vi "Catalytic Methanation #1.vi"() -> ()   [LabVIEW 2017]
uses:
  Halt S&THx.vi
  <vilib>/addons/control/pid/pid.llb/PID Advanced (DBL).vi
  <vilib>/addons/control/pid/NI_PID_pid.lvlib
panel:
  out "Heater Power Confirmed":bool
  in  "Td (Pressure)":dbl
  in  "Ti (Pressure)":dbl=0.01
  in  "Kc (Pressure)":dbl=-5.0
  in  "Td (Heater)":dbl caption="(min)"
  in  "Ti (Heater)":dbl=5.0 caption="(min)"
  in  "Kc (Heater)":dbl=1.0
  in  "GC Sample Path":enum32{"Reactor Feed", "Reactor Exhaust"}(radio)=enum."Reactor Exhaust"
  out "He Flowrate (SCCM)":dbl format="%.1f"
  out "H2 Flowrate (SCCM)":dbl format="%.2f"
  out "CO2 Flowrate (SCCM)":dbl format="%.2f"
  in  "He Setpoint (SCCM)":dbl min=0.0 max=200.0 format="%.1f"
  in  "H2 Setpoint (SCCM)":dbl min=0.0 max=50.0 format="%.2f"
  in  "Heater Switch":bool
  in  "CO2 Setpoint (SCCM)":dbl min=0.0 max=10.0 format="%.2f"
  in  "Temperature Setpoint (C)":dbl=20.0 min=0.0 max=325.0 format="%.1f"
  out "Reator Temperature (C)":dbl format="%.2f"
  out "Heater Output (%)":dbl(slide) scale=0.0..100.0
  in  "Manual Control Override (Temperature)":bool=TRUE
  in  "Set Manual Valve Heater Output (Temperature)":dbl(slide) scale=0.0..100.0
  in  "Reactor Pressure  Setpoint (psia)":dbl=18.4 min=0.0 max=30.0 format="%.1f"
  out "Reactor Pressure (psia)":dbl format="%.1f"
  out "Pressure Control Valve (%)":dbl(slide) scale=0.0..100.0
  in  "Manual Control Override (Pressure)":bool=TRUE
  in  "Set Manual Valve Position (Pressure)":dbl(slide)=50.0 scale=0.0..100.0
  in  "stop":bool
  out "Data Point Count":i32
  in  "Specify Time between Data Points (sec)":dbl=1.0
  in  "Cancel Data Collection":bool
  in  "Specify number of data points":i16=1
  in  "Enable 4":bool
  out "Saving Data 4":bool
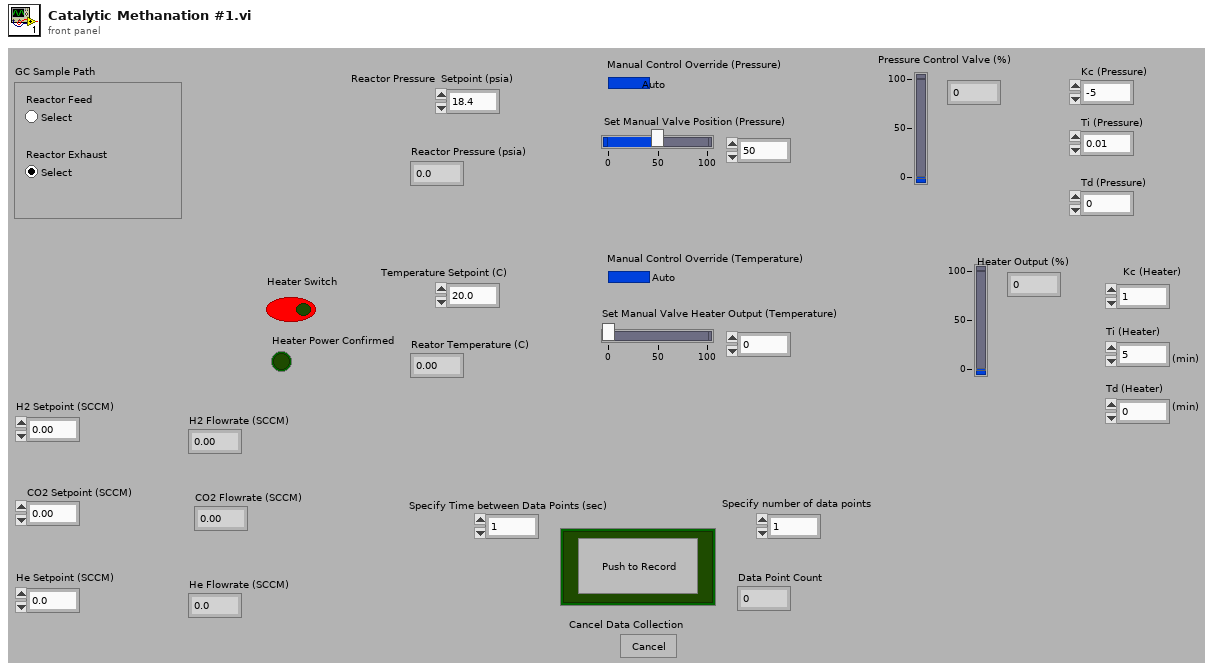
[diagram p1: front panel]
types:
  T1 = cluster{"Kc (Heater)":dbl, "Ti (Heater)":dbl, "Td (Heater)":dbl}
  T2 = cluster{"Kc (Pressure)":dbl, "Ti (Pressure)":dbl, "Td (Pressure)":dbl}
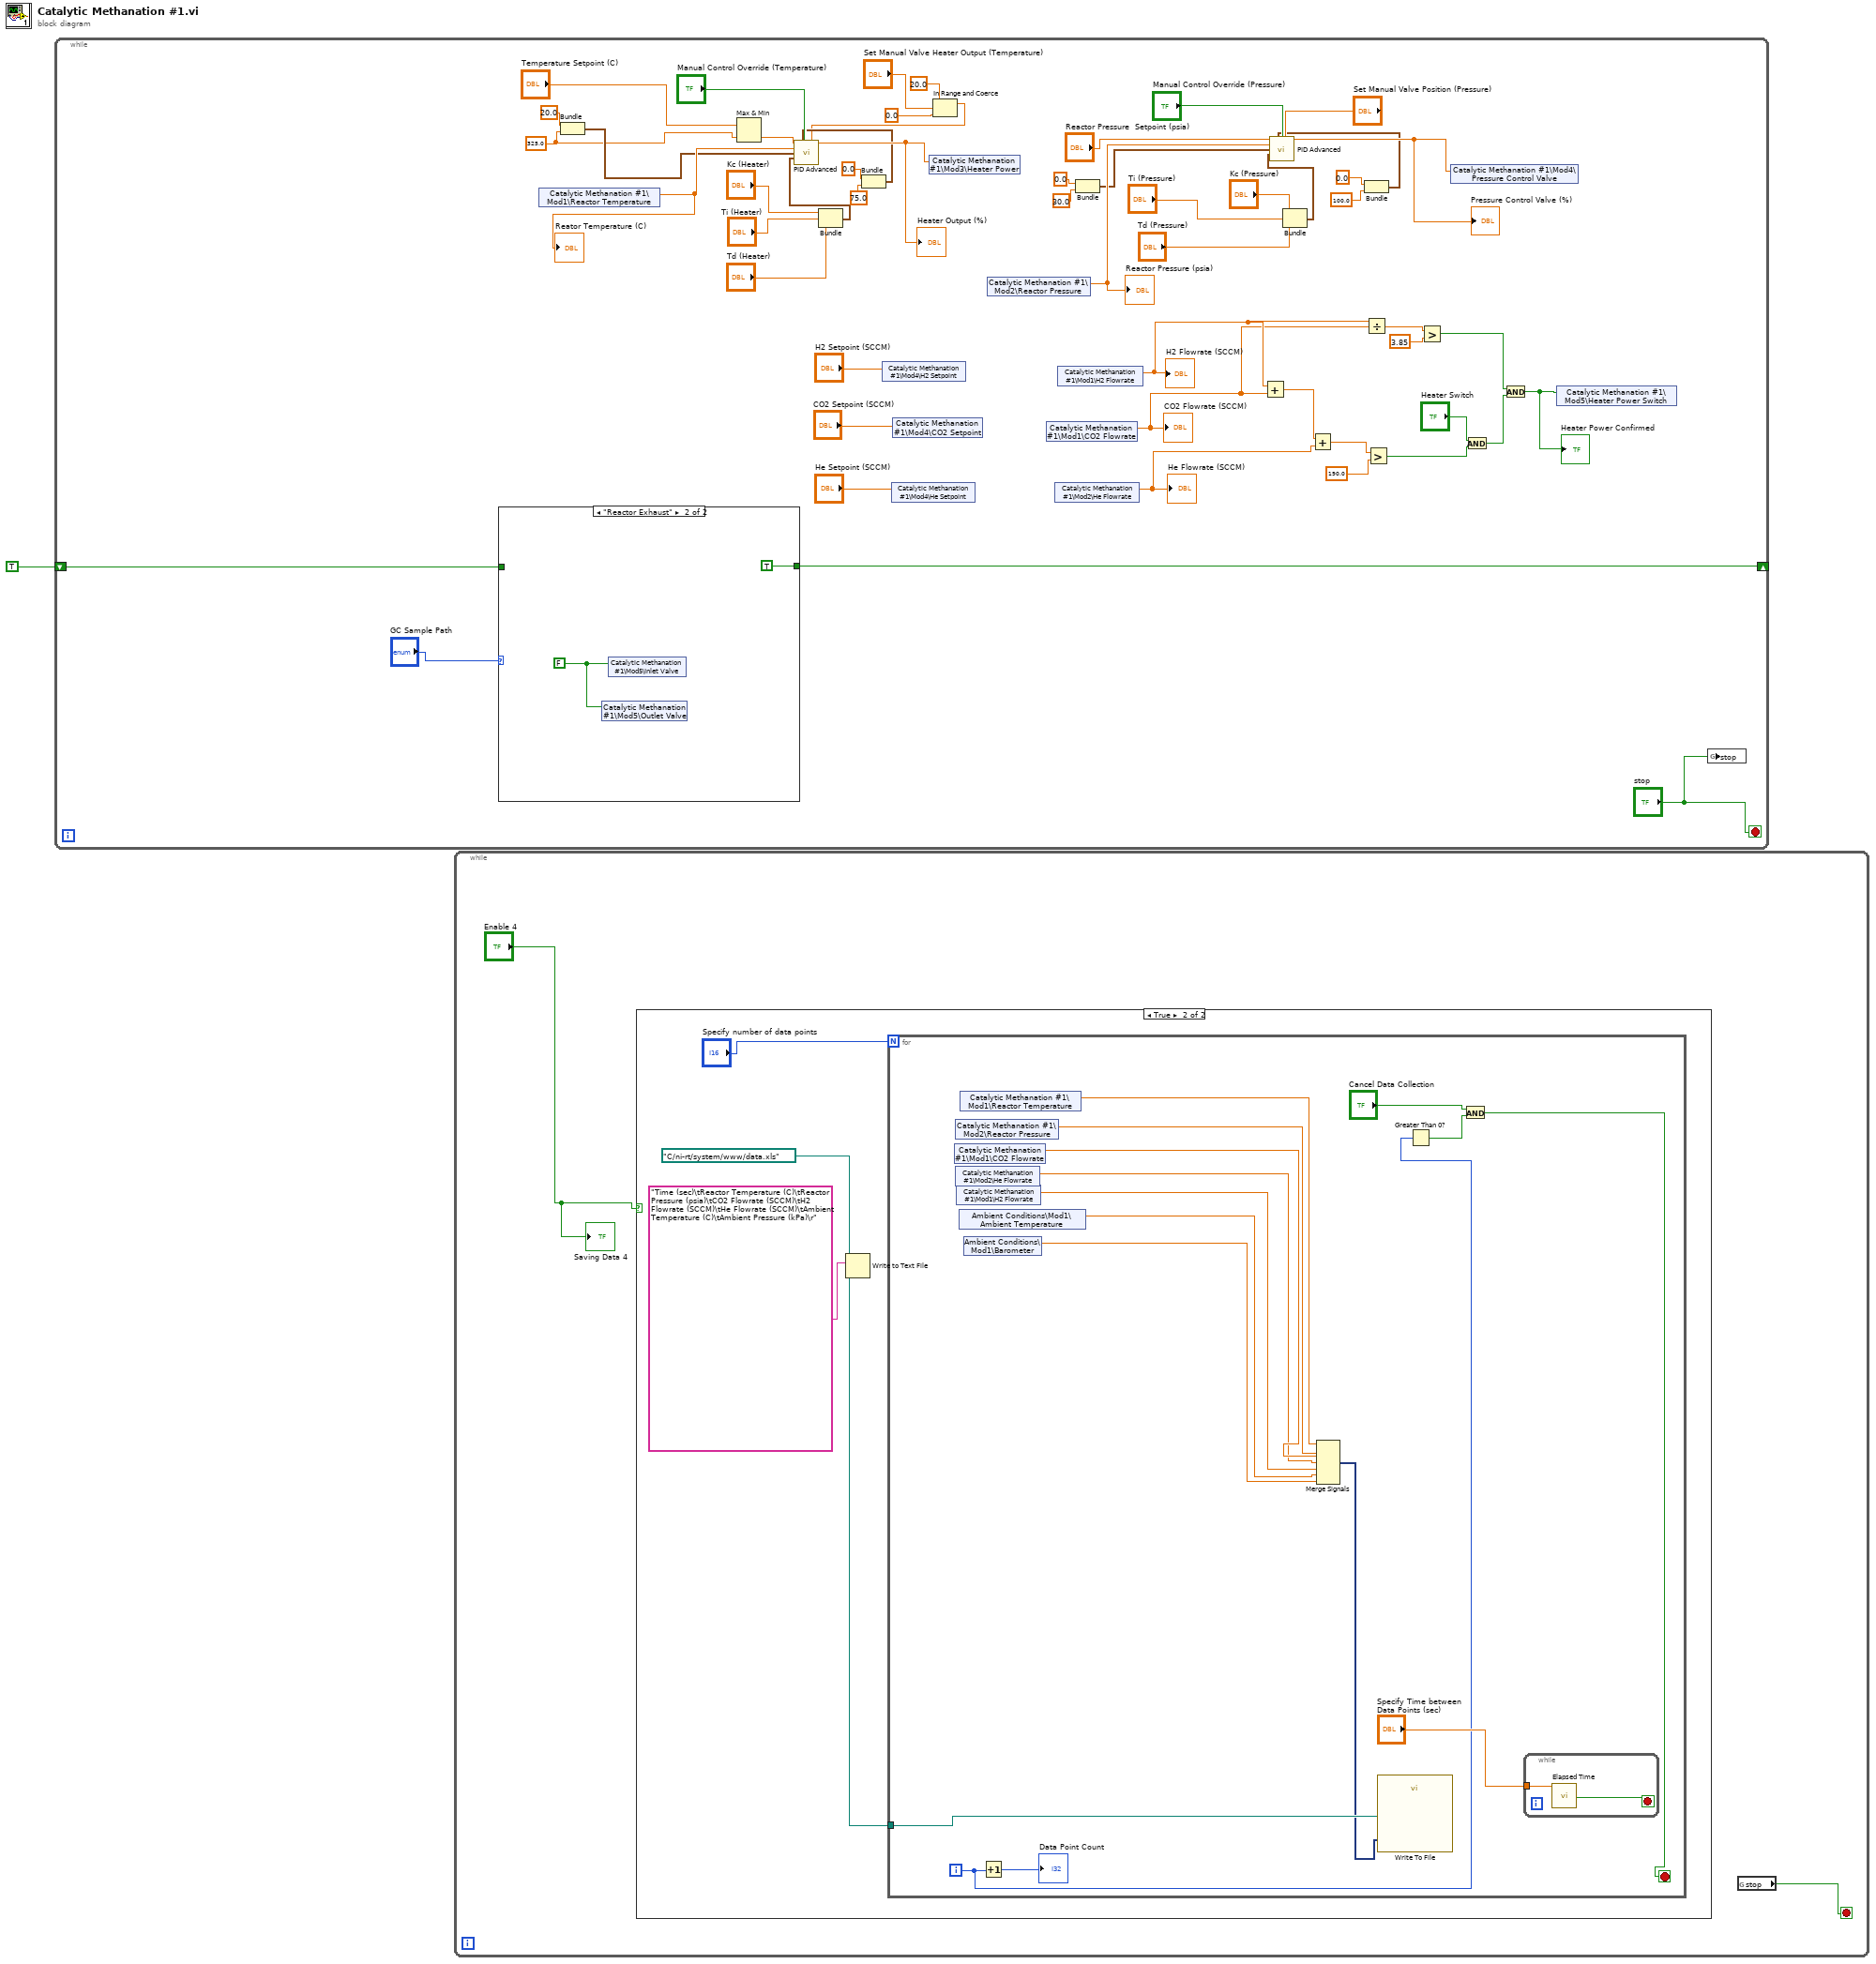
[diagram p0: block diagram]
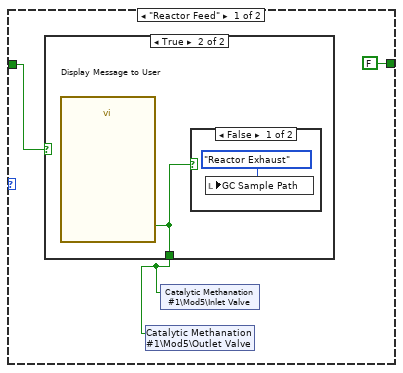
[diagram p2: hidden frame]
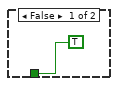
[diagram p3: hidden frame]
diagram:
  n1 = while {
    shift-right: [w9] -> _
    shift-left: TRUE -> [w10]
    stop <- "stop" stop-if-true
    w30 = 325.0
    n2 = case shown="\"Reactor Exhaust\"" "GC Sample Path" {
      tunnel: w10 -> [w56 _]
      tunnel: [FALSE TRUE] -> w9
      frame "Reactor Feed" {
        n3 = case shown="True" w56 {
          tunnel: [TRUE ("OK") w60] -> w58
          frame False {
          }
          frame True {
            n4 = call "Display Message to User"() -> ("OK"=w60:bool)  [unwired: 10 in, 1 out]
            n5 = case shown="False" w60 {
              frame False {
                n6 = local write "GC Sample Path"(enum32{"Reactor Feed", "Reactor Exhaust"}."Reactor Exhaust" ("GC Sample Path")) -> ()
              }
              frame True {
              }
            }
          }
        }
        n7 = shared-variable "Catalytic Methanation #1\\Mod5\\Outlet Valve"(w58) -> ()  [unwired: 1 in, 1 out]
        n8 = shared-variable "Catalytic Methanation #1\\Mod5\\Inlet Valve"(w58) -> ()  [unwired: 1 in, 1 out]
      }
      frame "Reactor Exhaust" {
        w63 = FALSE
        n9 = shared-variable "Catalytic Methanation #1\\Mod5\\Outlet Valve"(w63) -> ()  [unwired: 1 in, 1 out]
        n10 = shared-variable "Catalytic Methanation #1\\Mod5\\Inlet Valve"(w63) -> ()  [unwired: 1 in, 1 out]
      }
    }
    n11 = shared-variable "Catalytic Methanation #1\\Mod1\\Reactor Temperature"() -> (w41:dbl)  [unwired: 1 in, 1 out]
    "Reator Temperature (C)" <- w41
    n12 = Bundle(20.0, w30) -> (w32:cluster{dbl, dbl})  [unwired: 1 in]
    n13 = Max & Min(x="Temperature Setpoint (C)", y=w30) -> (min(x,y)=w22:dbl)  [unwired: 1 out]
    n14 = Bundle("Kc (Heater)"="Kc (Heater)", "Ti (Heater)"="Ti (Heater)", "Td (Heater)"="Td (Heater)") -> (w50:T1)  [unwired: 1 in]
    n15 = Bundle(0.0, 75.0) -> (w34:cluster{dbl, dbl})  [unwired: 1 in]
    n16 = shared-variable "Catalytic Methanation #1\\Mod4\\H2 Setpoint"("H2 Setpoint (SCCM)") -> ()  [unwired: 1 in, 1 out]
    n17 = shared-variable "Catalytic Methanation #1\\Mod4\\He Setpoint"("He Setpoint (SCCM)") -> ()  [unwired: 1 in, 1 out]
    n18 = shared-variable "Catalytic Methanation #1\\Mod4\\CO2 Setpoint"("CO2 Setpoint (SCCM)") -> ()  [unwired: 1 in, 1 out]
    n19 = In Range and Coerce(upper limit=20.0, x="Set Manual Valve Heater Output (Temperature)", lower limit=0.0) -> (coerced(x)=w20:dbl)  [unwired: 1 out]
    n20 = call-poly <vilib>:"PID Advanced.vi"("setpoint"=w22, "output range"=w34, "auto? (T)"="Manual Control Override (Temperature)", "manual control"=w20, "process variable"=w41, "setpoint range"=w32, "PID gains"=w50) -> ("output"=w43:dbl)  [unwired: 7 in, 1 out]
    "Heater Output (%)" <- w43
    n21 = shared-variable "Catalytic Methanation #1\\Mod3\\Heater Power"(w43) -> ()  [unwired: 1 in, 1 out]
    n22 = shared-variable "Catalytic Methanation #1\\Mod2\\Reactor Pressure"() -> (w52:dbl)  [unwired: 1 in, 1 out]
    "Reactor Pressure (psia)" <- w52
    n23 = shared-variable "Catalytic Methanation #1\\Mod1\\CO2 Flowrate"() -> (w7:dbl)  [unwired: 1 in, 1 out]
    "CO2 Flowrate (SCCM)" <- w7
    n24 = shared-variable "Catalytic Methanation #1\\Mod2\\He Flowrate"() -> (w17:dbl)  [unwired: 1 in, 1 out]
    "He Flowrate (SCCM)" <- w17
    n25 = shared-variable "Catalytic Methanation #1\\Mod1\\H2 Flowrate"() -> (w8:dbl)  [unwired: 1 in, 1 out]
    "H2 Flowrate (SCCM)" <- w8
    n26 = Bundle(0.0, 30.0) -> (w28:cluster{dbl, dbl})  [unwired: 1 in]
    n27 = Add(x=w8, y=w7) -> (x+y=w16:dbl)
    n28 = Bundle("Kc (Pressure)"="Kc (Pressure)", "Ti (Pressure)"="Ti (Pressure)", "Td (Pressure)"="Td (Pressure)") -> (w51:T2)  [unwired: 1 in]
    n29 = Add(x=w16, y=w17) -> (x+y=w15:dbl)
    n30 = Bundle(0.0, 100.0) -> (w25:cluster{dbl, dbl})  [unwired: 1 in]
    n31 = call-poly <vilib>:"PID Advanced.vi"("setpoint"="Reactor Pressure  Setpoint (psia)", "output range"=w25, "auto? (T)"="Manual Control Override (Pressure)", "manual control"="Set Manual Valve Position (Pressure)", "process variable"=w52, "setpoint range"=w28, "PID gains"=w51) -> ("output"=w55:dbl)  [unwired: 7 in, 1 out]
    "Pressure Control Valve (%)" <- w55
    n32 = Divide(x=w8, y=w7) -> (x/y=w6:dbl)
    n33 = Greater?(x=w15, y=190.0) -> (0:w13:bool)
    n34 = Greater?(x=w6, y=3.85) -> (0:w3:bool)
    n35 = shared-variable "Catalytic Methanation #1\\Mod4\\Pressure Control Valve"(w55) -> ()  [unwired: 1 in, 1 out]
    n36 = And(x="Heater Switch", y=w13) -> (x .and. y?=w4:bool)
    n37 = And(x=w3, y=w4) -> (x .and. y?=w2:bool)
    "Heater Power Confirmed" <- w2
    n38 = shared-variable "Catalytic Methanation #1\\Mod5\\Heater Power Switch"(w2) -> ()  [unwired: 1 in, 1 out]
    n39 = global write "Halt S&THx.vi" "stop"("stop") -> ()
  }
  n40 = while {
    stop <- w64 stop-if-true
    n41 = case shown="True" "Enable 4" {
      frame False {
      }
      frame True {
        w67 = path "C:/ni-rt/system/www/data.xls" ("Filename")
        n42 = Write to Text File(file (use dialog)=w67, text="Time (sec)\tReactor Temperature (C)\tReactor Pressure (psia)\tCO2 Flowrate (SCCM)\tH2 Flowrate (SCCM)\tHe Flowrate (SCCM)\tAmbient Temperature (C)\tAmbient Pressure (kPa)\r") -> ()  [unwired: 2 in, 3 out]
        n43 = for {
          N: "Specify number of data points" -> [_]
          tunnel: w67 -> [w83]
          i -> [w77]
          stop <- w74 stop-if-true
          n44 = shared-variable "Catalytic Methanation #1\\Mod1\\CO2 Flowrate"() -> (w80:dbl)  [unwired: 1 in, 1 out]
          n45 = shared-variable "Catalytic Methanation #1\\Mod2\\Reactor Pressure"() -> (w81:dbl)  [unwired: 1 in, 1 out]
          n46 = shared-variable "Catalytic Methanation #1\\Mod2\\He Flowrate"() -> (w73:dbl)  [unwired: 1 in, 1 out]
          n47 = shared-variable "Catalytic Methanation #1\\Mod1\\H2 Flowrate"() -> (w72:dbl)  [unwired: 1 in, 1 out]
          n48 = shared-variable "Ambient Conditions\\Mod1\\Ambient Temperature"() -> (w70:dbl)  [unwired: 1 in, 1 out]
          n49 = shared-variable "Catalytic Methanation #1\\Mod1\\Reactor Temperature"() -> (w71:dbl)  [unwired: 1 in, 1 out]
          n50 = shared-variable "Ambient Conditions\\Mod1\\Barometer"() -> (w69:dbl)  [unwired: 1 in, 1 out]
          n51 = Increment(x=w77) -> (x+1=→"Data Point Count":i32)
          n52 = Merge Signals(w71, w81, w80, w73, w72, w70, w69) -> (w79:dynamicdata)
          n53 = call "Write To File"("Signals"=w79, "Filename"=w83) -> ()  [unwired: 15 in, 3 out]
          n54 = Greater Than 0?(x=w77) -> (x > 0?=w75:bool)
          n55 = And(x="Cancel Data Collection", y=w75) -> (x .and. y?=w74:bool)
          n56 = while {
            tunnel: "Specify Time between Data Points (sec)" -> [w84]
            stop <- w85 stop-if-true
            n57 = call "Elapsed Time"("Time Target (s)"=w84) -> ("Time has Elapsed"=w85:bool)  [unwired: 11 in, 7 out]
          }
        }
      }
    }
    n58 = global read "Halt S&THx.vi" "stop"() -> (w64:bool)
    "Saving Data 4" <- "Enable 4"
  }
